vi "VPA QC Volume Calibration.vi"(9 "DAQ Ref Cluster":T5, 10 "State In":T1) -> (2 "State IOut":T1)   [LabVIEW 2013]
uses:
  Controls/VPA QC DAQ Ref Cluster.ctl
  Controls/VPA QC Scale Communication Settings DVR.ctl
  Controls/VPA QC Scale Communication Settings.ctl
  Controls/VPA QC State Data Cluster.ctl
  Controls/VPA QC General Cluster.ctl
  Controls/VPA QC State Enum.ctl
  Controls/VPA QC Bool Cluster.ctl
  Controls/VPA QC Vol Cal Data Cluster.ctl
panel:
  in  "Cancel":bool
  in  "Save":bool
  in  "A Side Calibration Constant":dbl caption="Flow Rate (mL/min)"
  in  "B Side Calibration Constant":dbl caption="Flow Rate (mL/min)"
  out "Average Difference 2":dbl caption="Average Difference" format="%#.5g"
  in  "Set Vol 6":bool
  in  "Set Vol 5":bool
  in  "Set Vol 4":bool
  in  "Volume to Flow 2":dbl=18.0 caption="Volume to Flow" step=0.1 format="%#_4g"
  out "Average 2":dbl caption="Average" format="%#.5g"
  out "% Difference 6":dbl format="%#.5g"
  out "% Difference 5":dbl format="%#.5f"
  out "% Difference 4":dbl caption="% Difference" format="%#.5f"
  out "Volume Measured 6":dbl
  out "Volume Measured 5":dbl
  out "Measured Volume 4":dbl caption="Current Vol \n(Mass/Density)"
  out "Average Difference":dbl format="%#.5g"
  in  "Set Vol 3":bool
  in  "Set Vol 2":bool
  in  "Set Vol 1":bool
  in  "Density of Fluid":dbl=0.996
  in  "Volume to Flow":dbl=18.0 step=0.1 format="%#_4g"
  out "Average":dbl format="%#.5g"
  out "% Difference 3":dbl format="%#.5g"
  out "% Difference 2":dbl format="%#.5f"
  out "% Difference 1":dbl caption="% Difference" format="%#.5f"
  out "Volume Measured 3":dbl
  out "Volume Measured 2":dbl
  out "Volume\nMeasured 1":dbl caption="Current Vol \n(Mass/Density)"
  # "Volume Calibration"
  # "Obtain graduated cylinders of 10 mL, 250 mL, and the size required for a full stroke for one cylinder.  Make sure that line is completely filled and there are no air bubbles.  Calibrate each cylinder through the following method for each cylinder:"
  # "1. Have a small reservoir to pull in fluid from either the outlet or inlet\n2. Fill the cylinder.\n3. Flow a full stroke onto the scale 3 times.  Record the data."
  # "A Side"
  # "B Side"
  # "5. In the terminal select actual measured and type in the average value and calculate new volume constant"
  # "Assembly Checklist"
  # "Assembly Checklist"
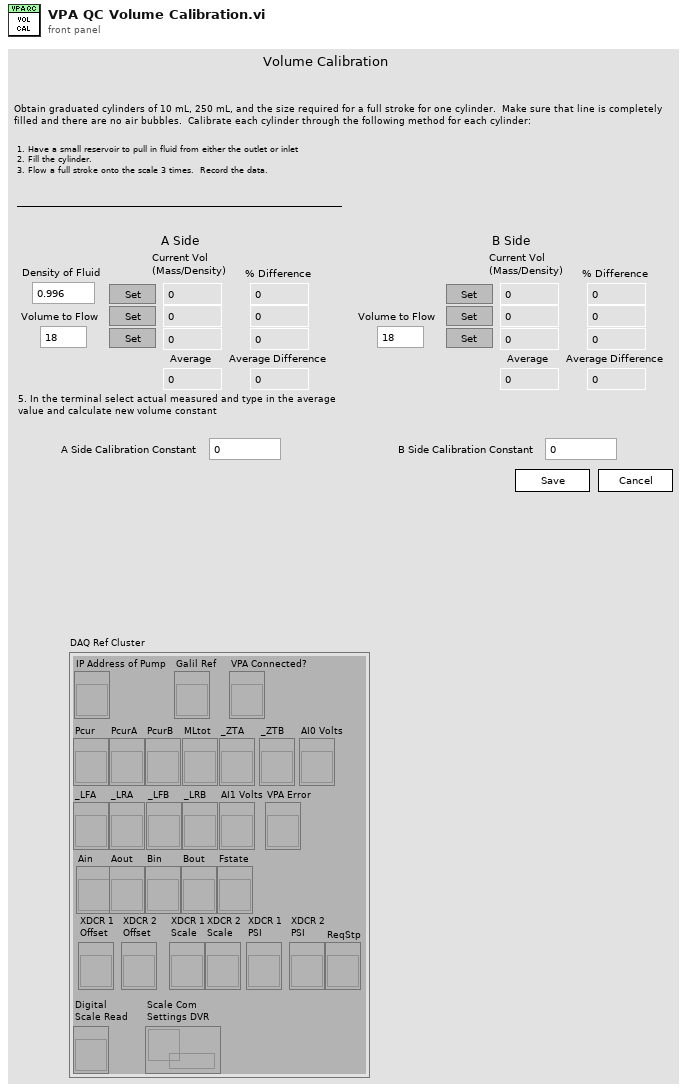
[diagram p1: front panel]
types:
  T1 = typedef "VPA QC State Data Cluster.ctl" = cluster{"XDCR 1":tag, "XDCR 2":tag, "General Information Clust":T2, "Assembly Checklist":cluster{"Ensure Drive Assembly checklist is completed.":bool, "Tighten Screws":bool, "Ensure VPA is wired correctly.":bool, "Ensure pump is running at voltage specified by customer.":bool}, "State":T3, "Manifold Leak Test Data":dbl[][], "Pressure Verification Test Data":dbl[][], "Flow Mode Verification Data":dbl[][], "DAQmx Error":errorcluster, "Bool Cluster":T4, "Leak Test Start Time":timestamp, "Pressure Test Start Time":timestamp, "Flow Test Start Time":timestamp, "Final Checklist cluster":cluster{"Check Fact Rest":bool, "Initialize Pump":bool, "Maintenance Hours":bool, "Clean Water Out":bool, "Covers":bool, "Screws":bool, "Wrap":bool, "Box":bool}, "Volts Constant":dbl, "Volume Constant A":dbl, "Volume Constant B":dbl, "Save File Path":path, "Comments Array":string[][], "File Format Version":u16}
  T2 = typedef "VPA QC General Cluster.ctl" = cluster{"Tech Name":string, "Date":timestamp, "Customer":string, "VPA Model":string, "G-72 Software Version":string, "Galil SN":string, "Galil Software Version":string, "VPA SN":string, "Valve SN":string, "Side A Drive Module SN":string, "Side B Drive Module SN":string, "A Side Transducer SN":string, "B Side Transducer SN":string, "A Side Motor SN":string, "B Side Motor SN":string, "A Side Gear Reducer SN":string, "B Side Gear Reducer SN":string, "A Side Limit Switch SN":string, "B Side Limit Switch SN":string, "Pump Voltage":string}
  T3 = typedef "VPA QC State Enum.ctl" = enum16{"General Information", "XDCR and LS Check", "Check Pump Function", "Manifold/Cylinder Leak Test", "Exit"}
  T4 = typedef "VPA QC Bool Cluster.ctl" = cluster{"Assembly":bool, "Gen":bool, "XDCR and LS Setup":bool, "Verify Pump Operation":bool, "Leak Test":bool, "Calibrate XDCRs":bool, "P Mode Verify":bool, "F Mode Verify":bool, "Vol Calibration":bool, "Flow Rate Test":bool, "Final Checklist":bool}
  T5 = typedef "VPA QC DAQ Ref Cluster.ctl" = cluster{"IP Address of Pump":refnum<vi>, "Galil Ref":refnum<vi>, "VPA Connected?":refnum<vi>, "Pcur":refnum<vi>, "PcurA":refnum<vi>, "PcurB":refnum<vi>, "MLtot":refnum<vi>, "_LFA":refnum<vi>, "_LRA":refnum<vi>, "_LFB":refnum<vi>, "_LRB":refnum<vi>, "_ZTA":refnum<vi>, "_ZTB":refnum<vi>, "AI0 Volts":refnum<vi>, "AI1 Volts":refnum<vi>, "VPA Error":refnum<vi>, "Ain":refnum<vi>, "Aout":refnum<vi>, "Bin":refnum<vi>, "Bout":refnum<vi>, "Fstate":refnum<vi>, "XDCR 1\nOffset":refnum<vi>, "XDCR 2 \nOffset":refnum<vi>, "XDCR 1\nScale":refnum<vi>, "XDCR 2\nScale":refnum<vi>, "XDCR 1\nPSI":refnum<vi>, "XDCR 2\nPSI":refnum<vi>, "ReqStp":refnum<vi>, "Digital \nScale Read":refnum<vi>, "Scale Com\nSettings DVR":T6}
  T6 = typedef "VPA QC Scale Communication Settings DVR.ctl" = refnum<data-value>
  T7 = typedef "VPA QC Vol Cal Data Cluster.ctl" = cluster{"Volume Measured 1":dbl, "Volume Measured 2":dbl, "Volume Measured 3":dbl, "% Difference 1":dbl, "% Difference 2":dbl, "% Difference 3":dbl, "Average":dbl, "Volume to Flow":dbl, "Set Vol 1":bool, "Set Vol 2":bool, "Set Vol 3":bool, "Average Difference":dbl}
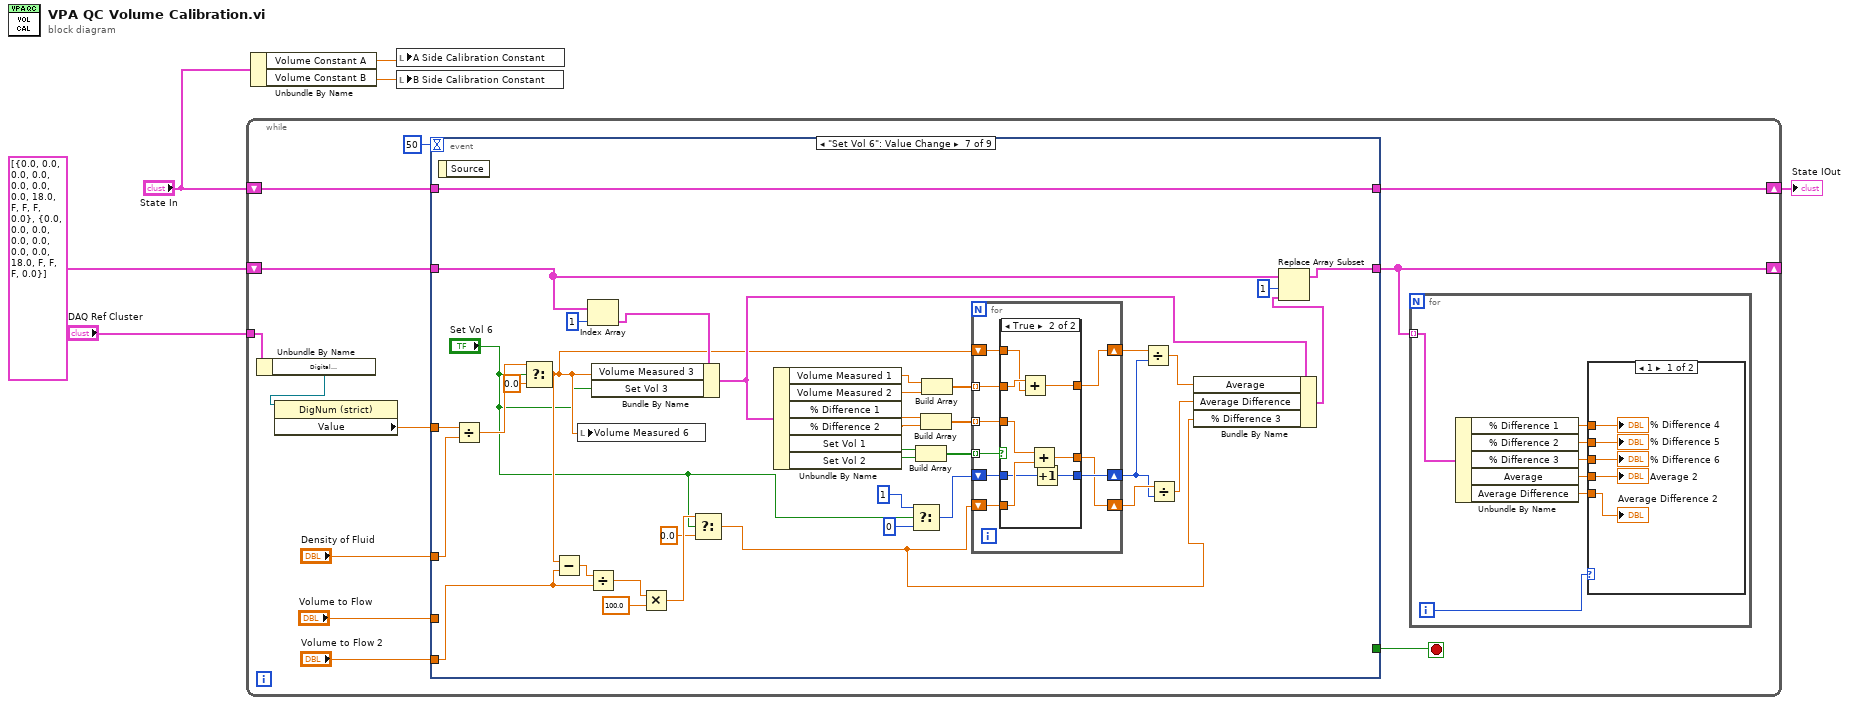
[diagram p0: block diagram]
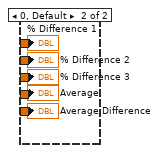
[diagram p2: hidden frame]
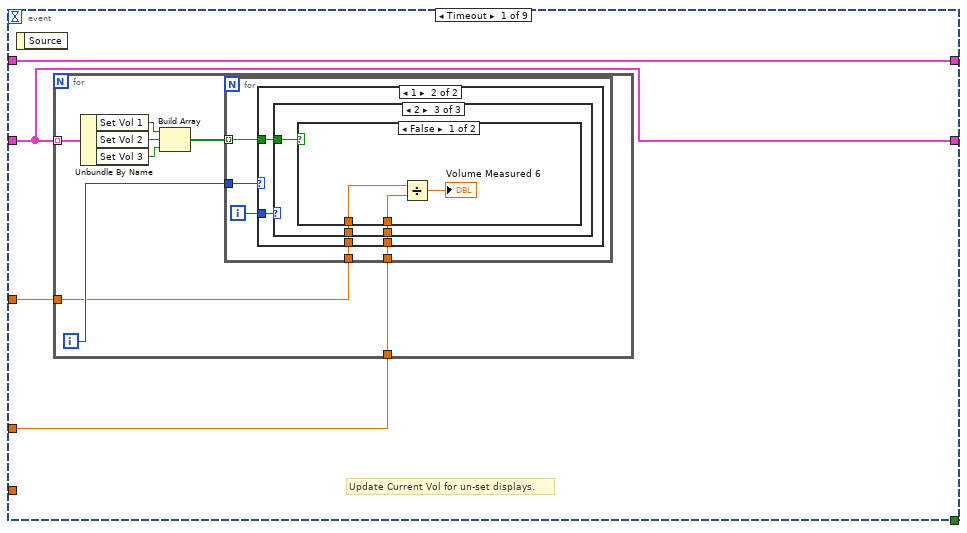
[diagram p3: hidden frame]
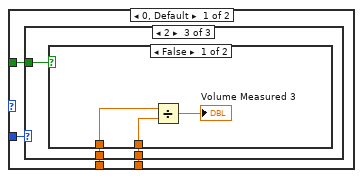
[diagram p4: hidden frame]
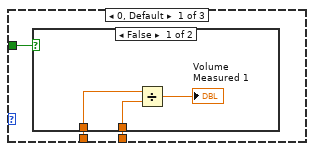
[diagram p5: hidden frame]
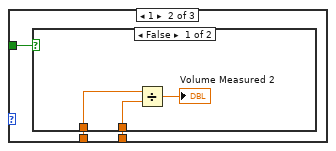
[diagram p7: hidden frame]
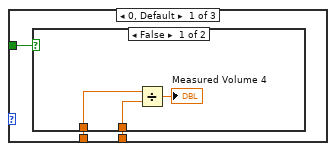
[diagram p10: hidden frame]
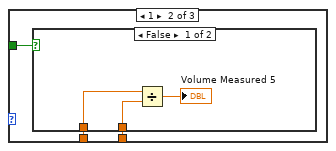
[diagram p12: hidden frame]
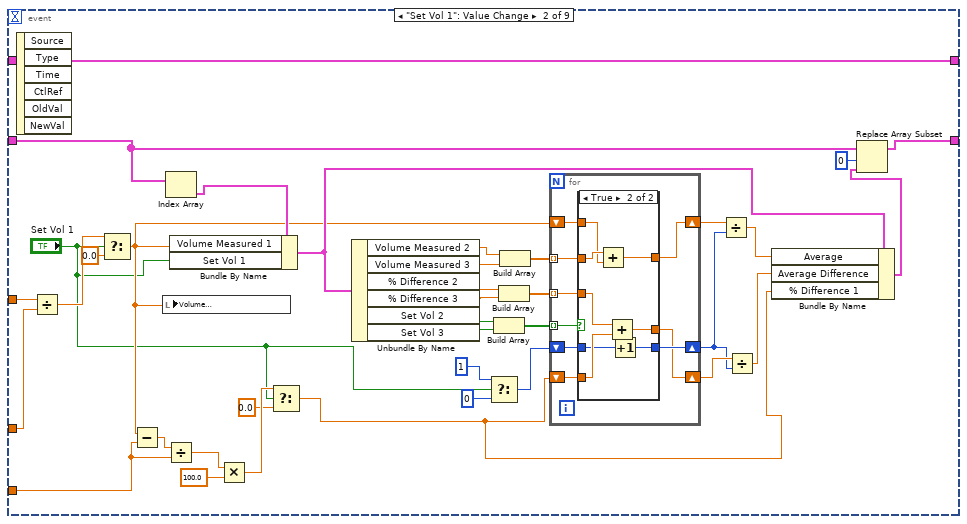
[diagram p15: hidden frame]
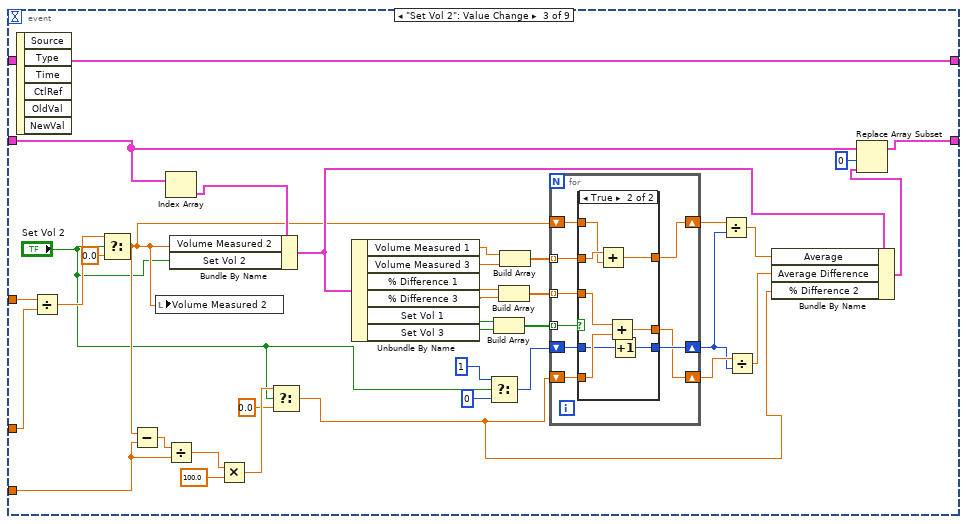
[diagram p17: hidden frame]
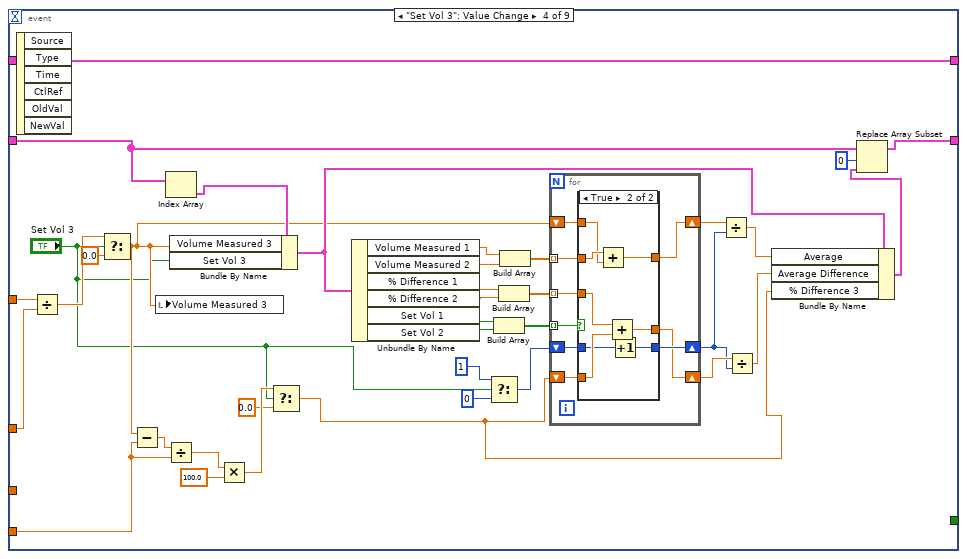
[diagram p19: hidden frame]
diagram:
  n1 = while {
    tunnel: "DAQ Ref Cluster" -> [w18]
    shift-right: [w10] -> _
    shift-left: T7[] [{"Volume Measured 1"=0.0, "Volume Measured 2"=0.0, "Volume Measured 3"=0.0, "% Difference 1"=0.0, "% Difference 2"=0.0, "% Difference 3"=0.0, "Average"=0.0, "Volume to Flow"=18.0, "Set Vol 1"=FALSE, "Set Vol 2"=FALSE, "Set Vol 3"=FALSE, "Average Difference"=0.0}, {"Volume Measured 1"=0.0, "Volume Measured 2"=0.0, "Volume Measured 3"=0.0, "% Difference 1"=0.0, "% Difference 2"=0.0, "% Difference 3"=0.0, "Average"=0.0, "Volume to Flow"=18.0, "Set Vol 1"=FALSE, "Set Vol 2"=FALSE, "Set Vol 3"=FALSE, "Average Difference"=0.0}] ("Cyl Vol Data Array") -> [w14]
    shift-right: [w7] -> w1
    shift-left: "State In" -> [w8]
    stop <- w12 stop-if-true
    n2 = Unbundle By Name(w18) -> ("Digital \nScale Read"=w17:refnum<vi>)
    n3 = property class="DigNum (strict)"(reference=w17) -> ("Value"=w15:dbl)  [unwired: 1 in, 2 out]
    n4 = event shown="[6] \"Set Vol 6\": Value Change" {
      selector: _ -> [_ _ _ _ _ _ _ _ _]
      dyn-events: _ -> [_ _ _ _ _ _ _ _ _]
      timeout: 50 -> [_ _ _ _ _ _ _ _ _]
      tunnel: w15 -> [w38 w132 w189 w246 w304 w362 w420 _ _]
      tunnel: w14 -> [w39 w130 w187 w244 w302 w360 w418 w443 w450]
      tunnel: "Density of Fluid" -> [w37 w131 w188 w245 w303 w361 w419 _ _]
      tunnel: [_ _ _ _ _ _ _ TRUE TRUE] -> w12
      tunnel: [w39 w128 w185 w242 w300 w358 w416 w443 w450] -> w10
      tunnel: "Volume to Flow" -> [_ w126 w183 _ _ _ _ _ _]
      tunnel: "Volume to Flow 2" -> [_ _ _ w211 w268 w326 w384 _ _]
      tunnel: w8 -> [w36 w97 w154 w212 w269 w328 w386 w442 w446]
      tunnel: [w36 w97 w154 w212 w269 w328 w386 w442 w445] -> w7
      event Timeout {
        # "Update Current Vol for un-set displays."
        n5 = event-data() -> ()  [unwired: 1 in, 1 out]
        n6 = for {
          tunnel: w39 -> [w47] mode=indexing
          tunnel: w38 -> [w41]
          tunnel: w37 -> [w40]
          i -> [w42]
          n7 = Unbundle By Name(w47) -> ("Set Vol 1"=w46:bool, "Set Vol 2"=w45:bool, "Set Vol 3"=w44:bool)
          n8 = Build Array(w46, w45, w44) -> (w43:bool[])
          n9 = for {
            tunnel: w43 -> [w50] mode=indexing
            tunnel: w42 -> [w52]
            tunnel: w41 -> [w49]
            tunnel: w40 -> [w48]
            i -> [w51]
            n10 = case shown="1" w52 {
              tunnel: w51 -> [w56 w78]
              tunnel: w50 -> [w55 w77]
              tunnel: w49 -> [w54 w76]
              tunnel: w48 -> [w53 w75]
              frame 0, Default {
                n11 = case shown="2" w56 {
                  tunnel: w55 -> [w59 w65 w71]
                  tunnel: w54 -> [w58 w64 w70]
                  tunnel: w53 -> [w57 w63 w69]
                  frame 0, Default {
                    n12 = case shown="False" w59 {
                      tunnel: w58 -> [w62 _]
                      tunnel: w57 -> [w61 _]
                      frame False {
                        n13 = Divide(x=w62, y=w61) -> (x/y=→"Volume\nMeasured 1":dbl)
                      }
                      frame True {
                      }
                    }
                  }
                  frame 1 {
                    n14 = case shown="False" w65 {
                      tunnel: w64 -> [w68 _]
                      tunnel: w63 -> [w67 _]
                      frame False {
                        n15 = Divide(x=w68, y=w67) -> (x/y=→"Volume Measured 2":dbl)
                      }
                      frame True {
                      }
                    }
                  }
                  frame 2 {
                    n16 = case shown="False" w71 {
                      tunnel: w70 -> [w74 _]
                      tunnel: w69 -> [w73 _]
                      frame False {
                        n17 = Divide(x=w74, y=w73) -> (x/y=→"Volume Measured 3":dbl)
                      }
                      frame True {
                      }
                    }
                  }
                }
              }
              frame 1 {
                n18 = case shown="2" w78 {
                  tunnel: w77 -> [w81 w87 w93]
                  tunnel: w76 -> [w80 w86 w92]
                  tunnel: w75 -> [w79 w85 w91]
                  frame 0, Default {
                    n19 = case shown="False" w81 {
                      tunnel: w80 -> [w84 _]
                      tunnel: w79 -> [w83 _]
                      frame False {
                        n20 = Divide(x=w84, y=w83) -> (x/y=→"Measured Volume 4":dbl)
                      }
                      frame True {
                      }
                    }
                  }
                  frame 1 {
                    n21 = case shown="False" w87 {
                      tunnel: w86 -> [w90 _]
                      tunnel: w85 -> [w89 _]
                      frame False {
                        n22 = Divide(x=w90, y=w89) -> (x/y=→"Volume Measured 5":dbl)
                      }
                      frame True {
                      }
                    }
                  }
                  frame 2 {
                    n23 = case shown="False" w93 {
                      tunnel: w92 -> [w96 _]
                      tunnel: w91 -> [w95 _]
                      frame False {
                        n24 = Divide(x=w96, y=w95) -> (x/y=→"Volume Measured 6":dbl)
                      }
                      frame True {
                      }
                    }
                  }
                }
              }
            }
          }
        }
      }
      event "Set Vol 1": Value Change {
        n25 = event-data() -> ()  [unwired: 1 in, 6 out]
        n26 = Divide(x=w132, y=w131) -> (x/y=w107:dbl)
        n27 = Select(t=w107, s="Set Vol 1", f=0.0) -> (s? t:f=w106:dbl)
        n28 = Subtract(x=w106, y=w126) -> (x-y=w127:dbl)
        n29 = local write "Volume\nMeasured 1"(w106) -> ()
        n30 = Index Array(array=w130) -> (element=w133:T7)  [unwired: 1 in]
        n31 = Divide(x=w127, y=w126) -> (x/y=w125:dbl)
        n32 = Bundle By Name(cluster=w133, "Volume Measured 1"=w106, "Set Vol 1"="Set Vol 1") -> (w111:T7)
        n33 = Multiply(x=w125, y=100.0) -> (x*y=w101:dbl)
        n34 = Select(t=w101, s="Set Vol 1", f=0.0) -> (s? t:f=w100:dbl)
        n35 = Unbundle By Name(w111) -> ("Volume Measured 2"=w116:dbl, "Volume Measured 3"=w115:dbl, "% Difference 2"=w120:dbl, "% Difference 3"=w119:dbl, "Set Vol 2"=w123:bool, "Set Vol 3"=w122:bool)
        n36 = Select(t=u8 1, s="Set Vol 1", f=u8 0) -> (s? t:f=w103:u8)
        n37 = Build Array(w123, w122) -> (w121:bool[])
        n38 = Build Array(w120, w119) -> (w118:dbl[])
        n39 = Build Array(w116, w115) -> (w114:dbl[])
        n40 = for {
          tunnel: w121 -> [w141] mode=indexing
          shift-right: [w138] -> w112
          shift-left: w103 -> [w142]
          tunnel: w118 -> [w140] mode=indexing
          shift-right: [w137] -> w117
          shift-left: w100 -> [w139]
          tunnel: w114 -> [w136] mode=indexing
          shift-right: [w134] -> w113
          shift-left: w106 -> [w135]
          n41 = case shown="True" w141 {
            tunnel: w142 -> [w145 w151]
            tunnel: w140 -> [_ w153]
            tunnel: w139 -> [w144 w152]
            tunnel: [w145 w150] -> w138
            tunnel: [w144 w149] -> w137
            tunnel: w136 -> [_ w148]
            tunnel: w135 -> [w143 w147]
            tunnel: [w143 w146] -> w134
            frame False {
            }
            frame True {
              n42 = Add(x=w148, y=w147) -> (x+y=w146:dbl)
              n43 = Add(x=w153, y=w152) -> (x+y=w149:dbl)
              n44 = Increment(x=w151) -> (x+1=w150:u8)
            }
          }
        }
        n45 = Divide(x=w113, y=w112) -> (x/y=w108:dbl)
        n46 = Divide(x=w117, y=w112) -> (x/y=w109:dbl)
        n47 = Bundle By Name(cluster=w111, "Average"=w108, "Average Difference"=w109, "% Difference 1"=w100) -> (w110:T7)
        n48 = Replace Array Subset(array=w130, new element=w110, index=0) -> (w128:T7[])
      }
      event "Set Vol 2": Value Change {
        n49 = event-data() -> ()  [unwired: 1 in, 6 out]
        n50 = Divide(x=w189, y=w188) -> (x/y=w164:dbl)
        n51 = Select(t=w164, s="Set Vol 2", f=0.0) -> (s? t:f=w163:dbl)
        n52 = Subtract(x=w163, y=w183) -> (x-y=w184:dbl)
        n53 = local write "Volume Measured 2"(w163) -> ()
        n54 = Index Array(array=w187) -> (element=w190:T7)  [unwired: 1 in]
        n55 = Divide(x=w184, y=w183) -> (x/y=w182:dbl)
        n56 = Bundle By Name(cluster=w190, "Volume Measured 2"=w163, "Set Vol 2"="Set Vol 2") -> (w168:T7)
        n57 = Multiply(x=w182, y=100.0) -> (x*y=w158:dbl)
        n58 = Select(t=w158, s="Set Vol 2", f=0.0) -> (s? t:f=w157:dbl)
        n59 = Unbundle By Name(w168) -> ("Volume Measured 1"=w173:dbl, "Volume Measured 3"=w172:dbl, "% Difference 1"=w177:dbl, "% Difference 3"=w176:dbl, "Set Vol 1"=w180:bool, "Set Vol 3"=w179:bool)
        n60 = Select(t=u8 1, s="Set Vol 2", f=u8 0) -> (s? t:f=w160:u8)
        n61 = Build Array(w180, w179) -> (w178:bool[])
        n62 = Build Array(w177, w176) -> (w175:dbl[])
        n63 = Build Array(w173, w172) -> (w171:dbl[])
        n64 = for {
          tunnel: w178 -> [w198] mode=indexing
          shift-right: [w195] -> w169
          shift-left: w160 -> [w199]
          tunnel: w175 -> [w197] mode=indexing
          shift-right: [w194] -> w174
          shift-left: w157 -> [w196]
          tunnel: w171 -> [w193] mode=indexing
          shift-right: [w191] -> w170
          shift-left: w163 -> [w192]
          n65 = case shown="True" w198 {
            tunnel: w199 -> [w202 w208]
            tunnel: w197 -> [_ w210]
            tunnel: w196 -> [w201 w209]
            tunnel: [w202 w207] -> w195
            tunnel: [w201 w206] -> w194
            tunnel: w193 -> [_ w205]
            tunnel: w192 -> [w200 w204]
            tunnel: [w200 w203] -> w191
            frame False {
            }
            frame True {
              n66 = Add(x=w205, y=w204) -> (x+y=w203:dbl)
              n67 = Add(x=w210, y=w209) -> (x+y=w206:dbl)
              n68 = Increment(x=w208) -> (x+1=w207:u8)
            }
          }
        }
        n69 = Divide(x=w170, y=w169) -> (x/y=w165:dbl)
        n70 = Divide(x=w174, y=w169) -> (x/y=w166:dbl)
        n71 = Bundle By Name(cluster=w168, "Average"=w165, "Average Difference"=w166, "% Difference 2"=w157) -> (w167:T7)
        n72 = Replace Array Subset(array=w187, new element=w167, index=0) -> (w185:T7[])
      }
      event "Set Vol 3": Value Change {
        n73 = event-data() -> ()  [unwired: 1 in, 6 out]
        n74 = Divide(x=w246, y=w245) -> (x/y=w222:dbl)
        n75 = Select(t=w222, s="Set Vol 3", f=0.0) -> (s? t:f=w221:dbl)
        n76 = Subtract(x=w221, y=w211) -> (x-y=w241:dbl)
        n77 = local write "Volume Measured 3"(w221) -> ()
        n78 = Index Array(array=w244) -> (element=w247:T7)  [unwired: 1 in]
        n79 = Divide(x=w241, y=w211) -> (x/y=w240:dbl)
        n80 = Bundle By Name(cluster=w247, "Volume Measured 3"=w221, "Set Vol 3"="Set Vol 3") -> (w226:T7)
        n81 = Multiply(x=w240, y=100.0) -> (x*y=w216:dbl)
        n82 = Select(t=w216, s="Set Vol 3", f=0.0) -> (s? t:f=w215:dbl)
        n83 = Unbundle By Name(w226) -> ("Volume Measured 1"=w231:dbl, "Volume Measured 2"=w230:dbl, "% Difference 1"=w235:dbl, "% Difference 2"=w234:dbl, "Set Vol 1"=w238:bool, "Set Vol 2"=w237:bool)
        n84 = Select(t=u8 1, s="Set Vol 3", f=u8 0) -> (s? t:f=w218:u8)
        n85 = Build Array(w238, w237) -> (w236:bool[])
        n86 = Build Array(w235, w234) -> (w233:dbl[])
        n87 = Build Array(w231, w230) -> (w229:dbl[])
        n88 = for {
          tunnel: w236 -> [w255] mode=indexing
          shift-right: [w252] -> w227
          shift-left: w218 -> [w256]
          tunnel: w233 -> [w254] mode=indexing
          shift-right: [w251] -> w232
          shift-left: w215 -> [w253]
          tunnel: w229 -> [w250] mode=indexing
          shift-right: [w248] -> w228
          shift-left: w221 -> [w249]
          n89 = case shown="True" w255 {
            tunnel: w256 -> [w259 w265]
            tunnel: w254 -> [_ w267]
            tunnel: w253 -> [w258 w266]
            tunnel: [w259 w264] -> w252
            tunnel: [w258 w263] -> w251
            tunnel: w250 -> [_ w262]
            tunnel: w249 -> [w257 w261]
            tunnel: [w257 w260] -> w248
            frame False {
            }
            frame True {
              n90 = Add(x=w262, y=w261) -> (x+y=w260:dbl)
              n91 = Add(x=w267, y=w266) -> (x+y=w263:dbl)
              n92 = Increment(x=w265) -> (x+1=w264:u8)
            }
          }
        }
        n93 = Divide(x=w228, y=w227) -> (x/y=w223:dbl)
        n94 = Divide(x=w232, y=w227) -> (x/y=w224:dbl)
        n95 = Bundle By Name(cluster=w226, "Average"=w223, "Average Difference"=w224, "% Difference 3"=w215) -> (w225:T7)
        n96 = Replace Array Subset(array=w244, new element=w225, index=0) -> (w242:T7[])
      }
      event "Set Vol 4": Value Change {
        n97 = event-data() -> ()  [unwired: 1 in, 1 out]
        n98 = Divide(x=w304, y=w303) -> (x/y=w280:dbl)
        n99 = Select(t=w280, s="Set Vol 4", f=0.0) -> (s? t:f=w279:dbl)
        n100 = Subtract(x=w279, y=w268) -> (x-y=w299:dbl)
        n101 = local write "Measured Volume 4"(w279) -> ()
        n102 = Index Array(array=w302, index=1) -> (element=w305:T7)
        n103 = Divide(x=w299, y=w268) -> (x/y=w298:dbl)
        n104 = Bundle By Name(cluster=w305, "Volume Measured 1"=w279, "Set Vol 1"="Set Vol 4") -> (w284:T7)
        n105 = Multiply(x=w298, y=100.0) -> (x*y=w274:dbl)
        n106 = Select(t=w274, s="Set Vol 4", f=0.0) -> (s? t:f=w273:dbl)
        n107 = Unbundle By Name(w284) -> ("Volume Measured 2"=w289:dbl, "Volume Measured 3"=w288:dbl, "% Difference 2"=w293:dbl, "% Difference 3"=w292:dbl, "Set Vol 2"=w296:bool, "Set Vol 3"=w295:bool)
        n108 = Select(t=u8 1, s="Set Vol 4", f=u8 0) -> (s? t:f=w276:u8)
        n109 = Build Array(w296, w295) -> (w294:bool[])
        n110 = Build Array(w293, w292) -> (w291:dbl[])
        n111 = Build Array(w289, w288) -> (w287:dbl[])
        n112 = for {
          tunnel: w294 -> [w313] mode=indexing
          shift-right: [w310] -> w285
          shift-left: w276 -> [w314]
          tunnel: w291 -> [w312] mode=indexing
          shift-right: [w309] -> w290
          shift-left: w273 -> [w311]
          tunnel: w287 -> [w308] mode=indexing
          shift-right: [w306] -> w286
          shift-left: w279 -> [w307]
          n113 = case shown="True" w313 {
            tunnel: w314 -> [w317 w323]
            tunnel: w312 -> [_ w325]
            tunnel: w311 -> [w316 w324]
            tunnel: [w317 w322] -> w310
            tunnel: [w316 w321] -> w309
            tunnel: w308 -> [_ w320]
            tunnel: w307 -> [w315 w319]
            tunnel: [w315 w318] -> w306
            frame False {
            }
            frame True {
              n114 = Add(x=w320, y=w319) -> (x+y=w318:dbl)
              n115 = Add(x=w325, y=w324) -> (x+y=w321:dbl)
              n116 = Increment(x=w323) -> (x+1=w322:u8)
            }
          }
        }
        n117 = Divide(x=w286, y=w285) -> (x/y=w281:dbl)
        n118 = Divide(x=w290, y=w285) -> (x/y=w282:dbl)
        n119 = Bundle By Name(cluster=w284, "Average"=w281, "Average Difference"=w282, "% Difference 1"=w273) -> (w283:T7)
        n120 = Replace Array Subset(array=w302, new element=w283, index=1) -> (w300:T7[])
      }
      event "Set Vol 5": Value Change {
        n121 = event-data() -> ()  [unwired: 1 in, 1 out]
        n122 = Divide(x=w362, y=w361) -> (x/y=w338:dbl)
        n123 = Select(t=w338, s="Set Vol 5", f=0.0) -> (s? t:f=w337:dbl)
        n124 = Subtract(x=w337, y=w326) -> (x-y=w357:dbl)
        n125 = local write "Volume Measured 5"(w337) -> ()
        n126 = Index Array(array=w360, index=1) -> (element=w363:T7)
        n127 = Divide(x=w357, y=w326) -> (x/y=w356:dbl)
        n128 = Bundle By Name(cluster=w363, "Volume Measured 2"=w337, "Set Vol 2"="Set Vol 5") -> (w342:T7)
        n129 = Multiply(x=w356, y=100.0) -> (x*y=w332:dbl)
        n130 = Select(t=w332, s="Set Vol 5", f=0.0) -> (s? t:f=w331:dbl)
        n131 = Unbundle By Name(w342) -> ("Volume Measured 1"=w347:dbl, "Volume Measured 3"=w346:dbl, "% Difference 1"=w351:dbl, "% Difference 3"=w350:dbl, "Set Vol 1"=w354:bool, "Set Vol 3"=w353:bool)
        n132 = Select(t=u8 1, s="Set Vol 5", f=u8 0) -> (s? t:f=w334:u8)
        n133 = Build Array(w354, w353) -> (w352:bool[])
        n134 = Build Array(w351, w350) -> (w349:dbl[])
        n135 = Build Array(w347, w346) -> (w345:dbl[])
        n136 = for {
          tunnel: w352 -> [w371] mode=indexing
          shift-right: [w368] -> w343
          shift-left: w334 -> [w372]
          tunnel: w349 -> [w370] mode=indexing
          shift-right: [w367] -> w348
          shift-left: w331 -> [w369]
          tunnel: w345 -> [w366] mode=indexing
          shift-right: [w364] -> w344
          shift-left: w337 -> [w365]
          n137 = case shown="True" w371 {
            tunnel: w372 -> [w375 w381]
            tunnel: w370 -> [_ w383]
            tunnel: w369 -> [w374 w382]
            tunnel: [w375 w380] -> w368
            tunnel: [w374 w379] -> w367
            tunnel: w366 -> [_ w378]
            tunnel: w365 -> [w373 w377]
            tunnel: [w373 w376] -> w364
            frame False {
            }
            frame True {
              n138 = Add(x=w378, y=w377) -> (x+y=w376:dbl)
              n139 = Add(x=w383, y=w382) -> (x+y=w379:dbl)
              n140 = Increment(x=w381) -> (x+1=w380:u8)
            }
          }
        }
        n141 = Divide(x=w344, y=w343) -> (x/y=w339:dbl)
        n142 = Divide(x=w348, y=w343) -> (x/y=w340:dbl)
        n143 = Bundle By Name(cluster=w342, "Average"=w339, "Average Difference"=w340, "% Difference 2"=w331) -> (w341:T7)
        n144 = Replace Array Subset(array=w360, new element=w341, index=1) -> (w358:T7[])
      }
      event "Set Vol 6": Value Change {
        n145 = event-data() -> ()  [unwired: 1 in, 1 out]
        n146 = Divide(x=w420, y=w419) -> (x/y=w396:dbl)
        n147 = Select(t=w396, s="Set Vol 6", f=0.0) -> (s? t:f=w395:dbl)
        n148 = Subtract(x=w395, y=w384) -> (x-y=w415:dbl)
        n149 = local write "Volume Measured 6"(w395) -> ()
        n150 = Index Array(array=w418, index=1) -> (element=w421:T7)
        n151 = Divide(x=w415, y=w384) -> (x/y=w414:dbl)
        n152 = Bundle By Name(cluster=w421, "Volume Measured 3"=w395, "Set Vol 3"="Set Vol 6") -> (w400:T7)
        n153 = Multiply(x=w414, y=100.0) -> (x*y=w390:dbl)
        n154 = Select(t=w390, s="Set Vol 6", f=0.0) -> (s? t:f=w389:dbl)
        n155 = Unbundle By Name(w400) -> ("Volume Measured 1"=w405:dbl, "Volume Measured 2"=w404:dbl, "% Difference 1"=w409:dbl, "% Difference 2"=w408:dbl, "Set Vol 1"=w412:bool, "Set Vol 2"=w411:bool)
        n156 = Select(t=u8 1, s="Set Vol 6", f=u8 0) -> (s? t:f=w392:u8)
        n157 = Build Array(w412, w411) -> (w410:bool[])
        n158 = Build Array(w409, w408) -> (w407:dbl[])
        n159 = Build Array(w405, w404) -> (w403:dbl[])
        n160 = for {
          tunnel: w410 -> [w429] mode=indexing
          shift-right: [w426] -> w401
          shift-left: w392 -> [w430]
          tunnel: w407 -> [w428] mode=indexing
          shift-right: [w425] -> w406
          shift-left: w389 -> [w427]
          tunnel: w403 -> [w424] mode=indexing
          shift-right: [w422] -> w402
          shift-left: w395 -> [w423]
          n161 = case shown="True" w429 {
            tunnel: w430 -> [w433 w439]
            tunnel: w428 -> [_ w441]
            tunnel: w427 -> [w432 w440]
            tunnel: [w433 w438] -> w426
            tunnel: [w432 w437] -> w425
            tunnel: w424 -> [_ w436]
            tunnel: w423 -> [w431 w435]
            tunnel: [w431 w434] -> w422
            frame False {
            }
            frame True {
              n162 = Add(x=w436, y=w435) -> (x+y=w434:dbl)
              n163 = Add(x=w441, y=w440) -> (x+y=w437:dbl)
              n164 = Increment(x=w439) -> (x+1=w438:u8)
            }
          }
        }
        n165 = Divide(x=w402, y=w401) -> (x/y=w397:dbl)
        n166 = Divide(x=w406, y=w401) -> (x/y=w398:dbl)
        n167 = Bundle By Name(cluster=w400, "Average"=w397, "Average Difference"=w398, "% Difference 3"=w389) -> (w399:T7)
        n168 = Replace Array Subset(array=w418, new element=w399, index=1) -> (w416:T7[])
      }
      event "Cancel": Value Change {
        n169 = event-data() -> ()  [unwired: 1 in, 1 out]
      }
      event "Save": Value Change {
        n170 = event-data() -> ()  [unwired: 1 in, 1 out]
        n171 = Bundle By Name(cluster=w446, "Volume Constant A"="A Side Calibration Constant", "Volume Constant B"="B Side Calibration Constant", "Bool Cluster.Vol Calibration"=TRUE) -> (w445:T1)
      }
    }
    n172 = for {
      tunnel: w10 -> [w25] mode=indexing
      i -> [w19]
      n173 = Unbundle By Name(w25) -> ("% Difference 1"=w24:dbl, "% Difference 2"=w23:dbl, "% Difference 3"=w22:dbl, "Average"=w21:dbl, "Average Difference"=w20:dbl)
      n174 = case shown="1" w19 {
        tunnel: w24 -> [w30 w35]
        tunnel: w23 -> [w28 w34]
        tunnel: w22 -> [w29 w33]
        tunnel: w21 -> [w27 w32]
        tunnel: w20 -> [w26 w31]
        frame 1 {
          "% Difference 4" <- w30
          "% Difference 5" <- w28
          "% Difference 6" <- w29
          "Average 2" <- w27
          "Average Difference 2" <- w26
        }
        frame 0, Default {
          "% Difference 1" <- w35
          "% Difference 2" <- w34
          "% Difference 3" <- w33
          "Average" <- w32
          "Average Difference" <- w31
        }
      }
    }
  }
  "State IOut" <- w1
  n175 = Unbundle By Name("State In") -> ("Volume Constant A"=w3:dbl, "Volume Constant B"=w2:dbl)
  n176 = local write "A Side Calibration Constant"(w3) -> ()
  n177 = local write "B Side Calibration Constant"(w2) -> ()
